vi "标准化长度.vi"(1 "原长度":i32) -> (0 "标准化长度":string)   [LabVIEW 2016, in "数据传输系统-06.lvlib" / "自动更新.lvlib" / "TCP文件传输系统.lvlib" / "TCP发送文件.lvlib"]
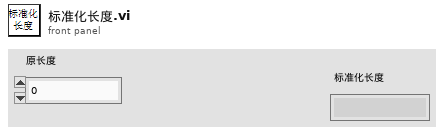
[diagram p1: front panel]
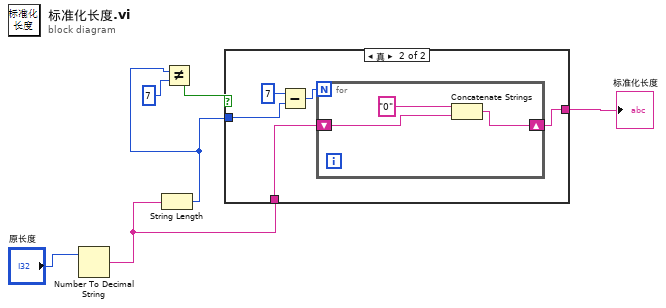
[diagram p0: block diagram]
diagram:
  n1 = Number To Decimal String(number="原长度") -> (decimal integer string=w1:string)  [unwired: 1 in]
  n2 = String Length(string=w1) -> (length=w4:i32)
  n3 = Not Equal?(x=w4, y=7 ("x")) -> (x != y?=w5:bool)
  n4 = case shown="真" w5 {
    tunnel: w4 -> [_ w12]
    tunnel: w1 -> [w7 w9]
    tunnel: [w7 w8] -> w3
    frame False {
    }
    frame True {
      n5 = Subtract(x=7, y=w12) -> (x-y=w10:i32)
      n6 = for {
        N: w10 -> [_]
        shift-right: [w14] -> w8
        shift-left: w9 -> [w13]
        n7 = Concatenate Strings("0", w13) -> (w14:string)
      }
    }
  }
  "标准化长度" <- w3
